vi "test1.vi"() -> ()   [LabVIEW 2022 SP3]
panel:
  out "String":string="import time\nimport ble_CBR\nimport bluetooth\nimport ble_advertising\nfrom ble_MIDI import *\nfrom hub import *\nimport device\nimport force_sensor\nimport distance_sensor\nimport motor\nimport color_sensor\nimport struct\nimport version\n\n\n#global\ndeviceTypeLookup = {48: 'm', 49: 'M', 61: 'Color S', 62: 'Distance S', 63: 'Force S', 255: 'N'}\nhubPorts = {'A': 'N', 'B': 'N', 'C': 'N', 'D': 'N', 'E': 'N', 'F': 'N'}\n\ndrumNotes = {31: 'Closed Hi-Hat', 32: 'Rim Shot', 33: 'Pedal Hi-Hat', 34: 'Snare Drum',\n    37: 'Side Stick', 39: 'Hand Clap', 41: 'Low Tom', 42: 'Closed Hi-Hat', 43: 'Low Tom',\n    44: 'Pedal Hi-Hat', 45: 'Mid Tom', 46: 'Open Hi-Hat', 47: 'Mid Tom', 48: 'High Tom',\n    49: 'Crash Cymbal', 50: 'High Tom', 51: 'Ride Cymbal', 52: 'Ride Cymbal', 53: 'Ride Bell',\n    54: 'Shaker', 57: 'Crash Cymbal', 59: 'Ride Cymbal', 86: 'Snare Drum', 90: 'Closed Hi-Hat',\n    91: 'Low Tom', 92: 'Closed Hi-Hat', 94: 'Pedal Hi-Hat', 95: 'Mid Tom',96: 'High Tom',\n    99: 'Ride Cymbal'}\n\n\n#initialize\nmidi = MIDI_Player('emma')\nmidi.wait_for_connection()\nPiano = MIDI_Instrument(midi, instruments['Acoustic Grand Piano'], channel=0)\n\n\n\n#firmware_check()\n\ndef done():\n    return button.pressed(button.RIGHT)\n\n\ndef test():\n    print(\"hi Emma!\")\n\n\ndef play_note(sensor, note, duration, dynamics = 'fff'):\n    \n    #print(\"in play_note\")\n\n    if type(note) == str:  \n        for key, value in drumNotes.items():\n            if value == note:\n                note = key  \n                #print(\"Found note:\", note)\n\n            \n    if (sensor == \"N\"):  \n        play_the_note(note, duration, dynamics)    \n        \n    elif (sensor == \"Force S\"):\n        if Force_Sensor_Activated():\n            play_the_note(note, duration, dynamics)\n        else:\n            print(\"waiing for FS activation\")\n            time.sleep(.1)\n            \n    elif (sensor == \"Color S\"):\n        if Color_Sensor_Activated():\n            play_the_note(note, duration, dynamics)\n        else:\n            print(\"waiting for CS activation\")\n            time.sleep(.1)\n            \n    elif (sensor == \"Distance S\"):\n        if Distance_Sensor_Activated():\n            the_port = check_port_connection(\"Distance S\")\n            dist = distance_sensor.distance(the_port)\n            dist_note = get_note_from_distance(dist)\n            play_the_note(dist_note, duration, dynamics)\n            #play_the_note(note, duration)\n        else:\n            print(\"waiting for DS activation\")\n            time.sleep(.1)\n            \n    elif ((sensor == \"m\") or (sensor == \"M\")):\n        #Need and if activated statment bc it could be not conencted\n        the_port = check_port_connection(sensor)\n        mpos = motor.absolute_position(the_port)\n    \n        if mpos < 0:\n            mpos = mpos + 360  \n        \n        print(mpos)\n        \n        note_range = 108 - 21  #Total number of notes in the range\n        note_value = int((mpos / 360) * note_range) + 21  #Maps the notes and value\n\n        play_the_note(note_value, .1, dynamics)\n        \n    else: \n        print(\"ELSE!!Invalid sensor type\")\n        time.sleep(.5)       \n\n\ndef play_chord(a, b=0, c=0, d=0, e=0, f=0, g=0, h=0):\n    Piano.on([a,b,c,d,e,f,g,h],velocity['f'])\n    time.sleep(.5)\n    Piano.off([a,b,c,d,e,f,g,h])\n        \n        \ndef play_the_note(note, duration, dynamics):\n    Piano.on(note, velocity[dynamics])\n    time.sleep(duration)\n    Piano.off(note, velocity[dynamics])\n\n\ndef Force_Sensor_Activated():\n    try:\n        the_port = check_port_connection(\"Force S\")\n        if the_port is None:\n            #print(\"Please connect the Force Sensor!\")\n            raise Exception(\"Force Sensor is NOT connected\")\n\n        if force_sensor.force(the_port) > 0:\n            print(\"Force Sensor is ACTIVATED\")\n            return True\n        else:\n            #print(\"FS FALSE\")\n            #time.sleep(.25)\n            return False\n    except Exception as e:\n        print(f\"Error: {e}\")\n        time.sleep(2)\n        return False\n    \ndef Color_Sensor_Activated():\n    try:\n        the_port = check_port_connection(\"Color S\")\n\n        if the_port is None:\n            #print(\"Please connect the Color Sensor!\")\n            raise Exception(\"Color Sensor is NOT connected\")\n\n        reflection = color_sensor.reflection(the_port)\n        if reflection > 50:\n            print(\"Color Sensor is ACTIVATED\")\n            return True\n        else:\n            return False\n    except Exception as e:\n        print(f\"Error: {e}\")\n        time.sleep(2)\n        return False\n    \n        \ndef Distance_Sensor_Activated():\n    try:\n        the_port = check_port_connection(\"Distance S\")\n        if the_port is None:\n            #print(\"Please connect the Distance Sensor!\")\n            raise Exception(\"Distance Sensor is NOT connected\")\n        \n        if distance_sensor.distance(the_port) > 0:\n            return True\n        else:\n            return False\n            \n    except Exception as e:\n        print(f\"Error: {e}\")\n        time.sleep(2)\n        return False    \n\n\n#def Motor_Activated():\n    \n\ndef disconnect():\n    print('disconnect')\n    midi.disconnect()\n\n\n\n\ndef NoteToNumber(note, octave = 0):\n    notes = {\"C\": 24,\"Db\": 25,\"D\": 26,\"Eb\": 27,\"E\": 28,\"F\": 29,\"Gb\": 30,\"G\": 31,\"Ab\": 32, \"A\": 33,\"Bb\": 34,\"B\": 35}\n    \n    try:  \n        if octave > 8 or octave < 0:\n            raise Exception(\"Invalid octave input\")\n        if note not in notes:\n            raise Exception(\"Invalid note input\")\n    \n        if(octave > 0):\n            return((notes[note]) + (octave*12))\n        \n    except Exception as e:\n        print(f\"Error: {e}\")\n        time.sleep(2)\n        return False\n        \n    \n'''-----Helper functions section (NOT intended for the user to use!)-----'''\n\ndef firmware_check():\n    try:\n        version.atlantis\n        print(version.atlantis)\n        print(\"Firmware is up to date! Good Job!\")\n    except:\n        print(\"Old Firmware: Please update your LEGO SPIKE hub to the latest firmware!\")\n\n\ndef get_note_from_distance(dist):\n    if dist == -1 or dist > 500:\n        return -1\n    elif dist < 500:\n        note = int(8 + (dist / 5))\n        return note\n\n\n\ndef ReadPorts():   \n    i = 0\n    for key in sorted(hubPorts): \n        hubPorts[key] = deviceTypeLookup.get(device.device_id(i))\n        i+=1\n            \n    return None\n\n\ndef is_connected(sensor):\n    ReadPorts()\n    \n    there_is_sensor = False\n    \n    i = 0\n    for port in sorted(hubPorts):\n        \n        if hubPorts[port] == sensor:\n            print(f\"{sensor} is connected to port.{port}\")\n            there_is_sensor = True\n    \n        if i == 5 and not there_is_sensor:\n            print(f\"{sensor} is NOT connected\")\n            print(\"--------------\")\n            raise ValueError(f\"{sensor} is not connected to any port\")\n            return False\n            \n        if i == 5 and there_is_sensor:\n            return True\n            \n        i+=1\n\n    return False\n\n\ndef check_port_connection(sensor):\n    ReadPorts()\n\n    i = 0\n    for port in sorted(hubPorts):\n        \n        if hubPorts[port] == sensor:\n            #print(\"connected\")\n            return string2port(f\"port.{port}\")\n            #return(f\"port.{port}\")\n    \n        if i == 5:\n            print(f\"{sensor} is NOT connected\")\n            print(\"--------------\")\n            #raise Exception(f\"{sensor} is NOT connected\")\n            return None\n    i+=1\n\n    return None\n        \n    \ndef string2port(portS):\n    if portS == \"port.A\": return port.A\n    if portS == \"port.B\": return port.B\n    if portS == \"port.C\": return port.C\n    if portS == \"port.D\": return port.D\n    if portS == \"port.E\": return port.E\n    if portS == \"port.F\": return port.F\n"
  out "number of replacements":i32
  out "result string":string
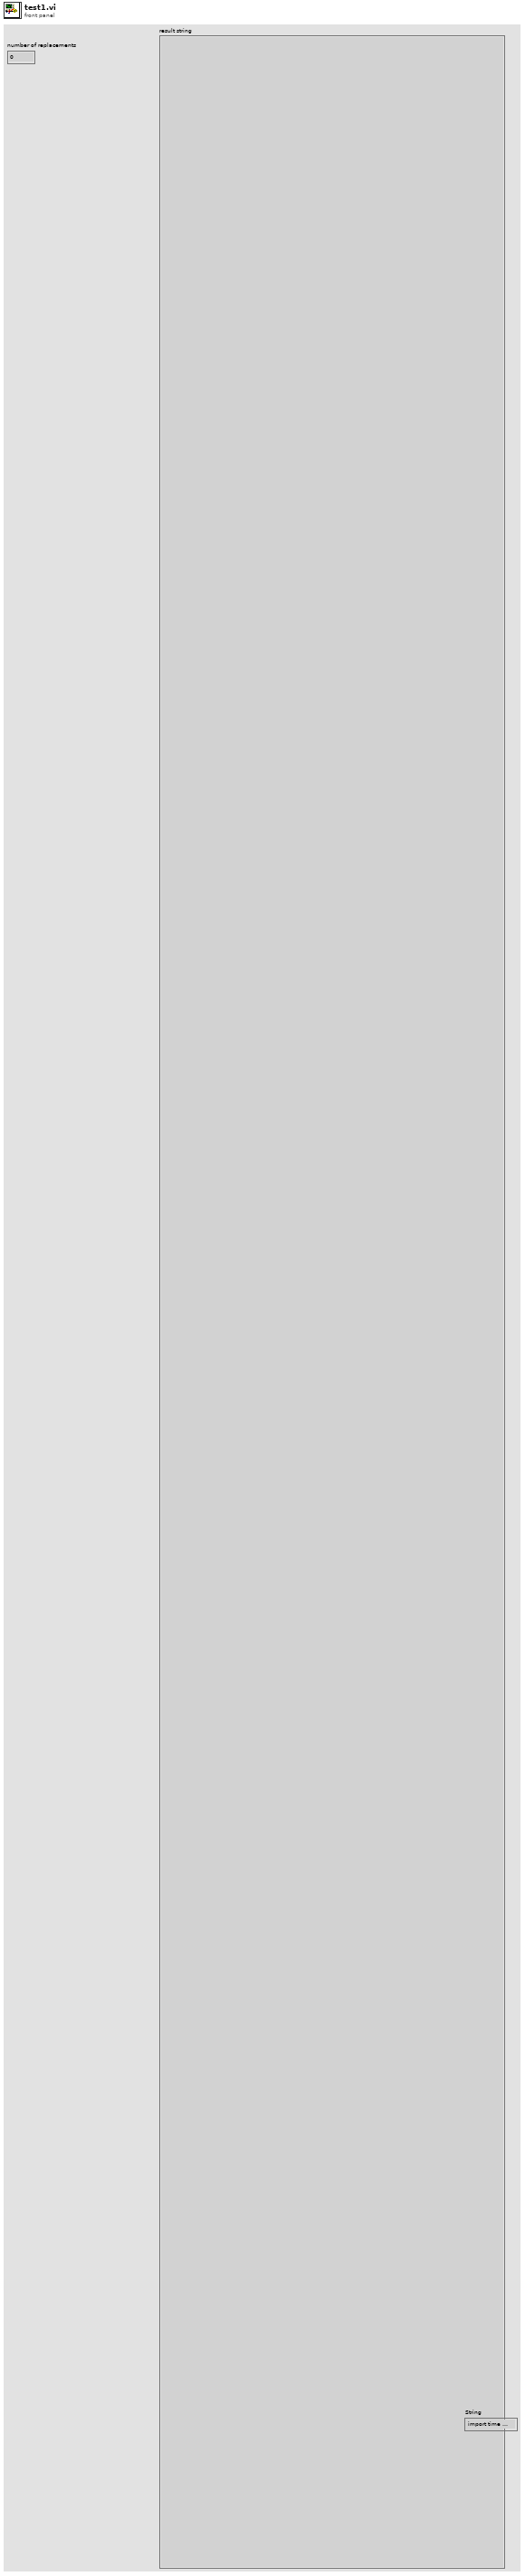
[diagram p1: front panel]
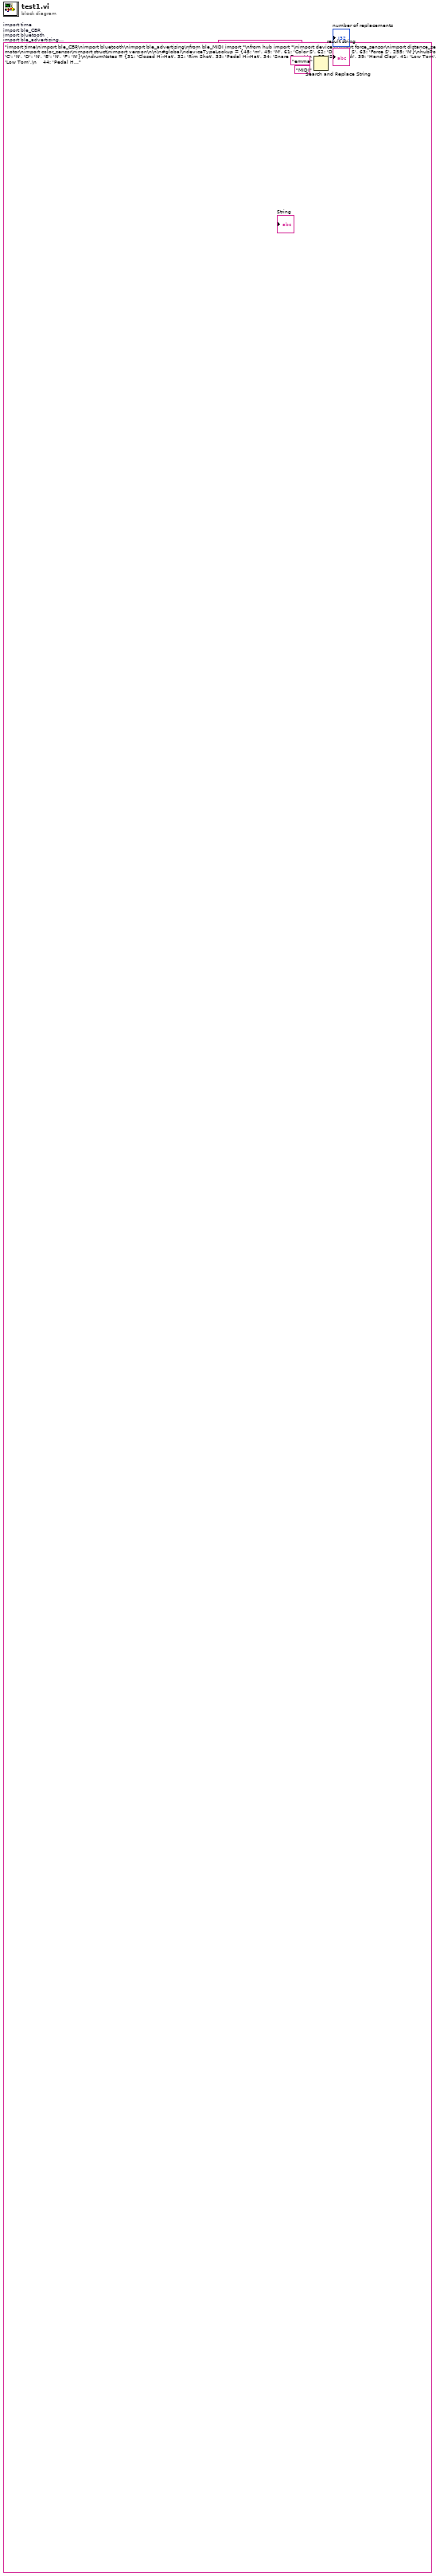
[diagram p0: block diagram]
diagram:
  w5 = "import time\nimport ble_CBR\nimport bluetooth\nimport ble_advertising\nfrom ble_MIDI import *\nfrom hub import *\nimport device\nimport force_sensor\nimport distance_sensor\nimport motor\nimport color_sensor\nimport struct\nimport version\n\n\n#global\ndeviceTypeLookup = {48: 'm', 49: 'M', 61: 'Color S', 62: 'Distance S', 63: 'Force S', 255: 'N'}\nhubPorts = {'A': 'N', 'B': 'N', 'C': 'N', 'D': 'N', 'E': 'N', 'F': 'N'}\n\ndrumNotes = {31: 'Closed Hi-Hat', 32: 'Rim Shot', 33: 'Pedal Hi-Hat', 34: 'Snare Drum',\n    37: 'Side Stick', 39: 'Hand Clap', 41: 'Low Tom', 42: 'Closed Hi-Hat', 43: 'Low Tom',\n    44: 'Pedal Hi-Hat', 45: 'Mid Tom', 46: 'Open Hi-Hat', 47: 'Mid Tom', 48: 'High Tom',\n    49: 'Crash Cymbal', 50: 'High Tom', 51: 'Ride Cymbal', 52: 'Ride Cymbal', 53: 'Ride Bell',\n    54: 'Shaker', 57: 'Crash Cymbal', 59: 'Ride Cymbal', 86: 'Snare Drum', 90: 'Closed Hi-Hat',\n    91: 'Low Tom', 92: 'Closed Hi-Hat', 94: 'Pedal Hi-Hat', 95: 'Mid Tom',96: 'High Tom',\n    99: 'Ride Cymbal'}\n\n\n#firmware_check()\n\ndef done():\n    return button.pressed(button.RIGHT)\n\n\ndef test():\n    print(\"hi Emma!\")\n\n\ndef play_note(sensor = \"N\", note = 60, duration = 1, dynamics = 'fff', port = None):\n    \n    #print(\"in play_note\")\n\n    if type(note) == str:  \n        for key, value in drumNotes.items():\n            if value == note:\n                note = key  \n                #print(\"Found note:\", note)\n\n            \n    if (sensor == \"N\"):  \n        play_the_note(note, duration, dynamics)    \n        \n    elif (sensor == \"Force S\"):\n        if Force_Sensor_Activated(port):\n            play_the_note(note, duration, dynamics)\n        else:\n            print(\"waiing for FS activation\")\n            time.sleep(.1)\n            \n    elif (sensor == \"Color S\"):\n        if Color_Sensor_Activated(port):\n            play_the_note(note, duration, dynamics)\n        else:\n            print(\"waiting for CS activation\")\n            time.sleep(.1)\n            \n    elif (sensor == \"Distance S\"):\n        if Distance_Sensor_Activated(port):\n            the_port = check_port_connection(\"Distance S\")\n            dist = distance_sensor.distance(the_port)\n            dist_note = get_note_from_distance(dist)\n            play_the_note(dist_note, duration, dynamics)\n            #play_the_note(note, duration)\n        else:\n            print(\"waiting for DS activation\")\n            time.sleep(.1)\n            \n    elif ((sensor == \"m\") or (sensor == \"M\")):\n        #Need and if activated statment bc it could be not conencted\n        the_port = check_port_connection(sensor)\n        mpos = motor.absolute_position(the_port)\n    \n        if mpos < 0:\n            mpos = mpos + 360  \n        \n        print(mpos)\n        \n        note_range = 108 - 21  #Total number of notes in the range\n        note_value = int((mpos / 360) * note_range) + 21  #Maps the notes and value\n\n        play_the_note(note_value, .1, dynamics)\n        \n    else: \n        print(\"ELSE!!Invalid sensor type\")\n        time.sleep(.5)       \n\n\ndef play_chord(a, b=0, c=0, d=0, e=0, f=0, g=0, h=0):\n    Piano.on([a,b,c,d,e,f,g,h],velocity['ff'])\n    time.sleep(.5)\n    Piano.off([a,b,c,d,e,f,g,h])\n        \n        \ndef play_the_note(note, duration, dynamics):\n    Piano.on(note, velocity[dynamics])\n    time.sleep(duration)\n    Piano.off(note, velocity[dynamics])\n\n\ndef Force_Sensor_Activated(port):\n    try:\n        if port is None:\n            the_ports = check_port_connection(\"Force S\")\n            if the_ports is None:\n                #print(\"Please connect the Force Sensor!\")\n                raise Exception(\"Force Sensor is NOT connected\")\n            \n            for port in the_ports:\n                if force_sensor.force(port) > 0:\n                    print(\"Force Sensor is ACTIVATED\")\n                    return True\n            \n            return False\n        else:\n            #print(\"Port was typed\") \n            if force_sensor.force(port) > 0:\n                print(\"Force Sensor is ACTIVATED\")\n                return True\n            else:\n                #print(\"FS FALSE\")\n                #time.sleep(.25)\n                return False\n                           \n    except Exception as e:\n        print(f\"Error: {e}\")\n        time.sleep(2)\n        return False\n\n\n    \ndef Color_Sensor_Activated(port):\n    try:\n        if port is None:\n            the_ports = check_port_connection(\"Color S\")\n            if the_ports is None:\n                #print(\"Please connect the Color Sensor!\")\n                raise Exception(\"Color Sensor is NOT connected\")\n            \n            for port in the_ports:\n                if color_sensor.reflection(port) > 50:\n                    print(\"Color Sensor is ACTIVATED\")\n                    return True\n            \n            return False\n        else:\n            if color_sensor.reflection(port) > 50:\n                print(\"Color Sensor is ACTIVATED\")\n                return True\n            else:\n                return False\n                \n    except Exception as e:\n        print(f\"Error: {e}\")\n        time.sleep(2)\n        return False\n  \n        \ndef Distance_Sensor_Activated(port):\n    try:\n        if port is None:\n            the_ports = check_port_connection(\"Distance S\")\n            if the_ports is None:\n                #print(\"Please connect the Color Sensor!\")\n                raise Exception(\"Distance Sensor is NOT connected\")\n            \n            for port in the_ports:\n                if distance_sensor.distance(the_port) > 0:\n                    print(\"Distance Sensor is ACTIVATED\")\n                    return True\n\n            return False\n        else:\n            if color_sensor.reflection(port) > 50:\n                print(\"Color Sensor is ACTIVATED\")\n                return True\n            else:\n                return False\n\n    except Exception as e:\n        print(f\"Error: {e}\")\n        time.sleep(2)\n        return False    \n\n\n#def Motor_Activated():\n    \n\ndef disconnect():\n    print('disconnect')\n    midi.disconnect()\n\n\n\n\ndef NoteToNumber(note, octave = 0):\n    notes = {\"C\": 24,\"Db\": 25,\"D\": 26,\"Eb\": 27,\"E\": 28,\"F\": 29,\"Gb\": 30,\"G\": 31,\"Ab\": 32, \"A\": 33,\"Bb\": 34,\"B\": 35}\n    \n    try:  \n        if octave > 8 or octave < 0:\n            raise Exception(\"Invalid octave input\")\n        if note not in notes:\n            raise Exception(\"Invalid note input\")\n    \n        if(octave > 0):\n            return((notes[note]) + (octave*12))\n        \n    except Exception as e:\n        print(f\"Error: {e}\")\n        time.sleep(2)\n        return False\n        \n    \n'''-----Helper functions section (NOT intended for the user to use!)-----'''\n\ndef firmware_check():\n    try:\n        version.atlantis\n        print(version.atlantis)\n        print(\"Firmware is up to date! Good Job!\")\n    except:\n        print(\"Old Firmware: Please update your LEGO SPIKE hub to the latest firmware!\")\n\n\ndef get_note_from_distance(dist):\n    if dist == -1 or dist > 500:\n        return -1\n    elif dist < 500:\n        note = int(8 + (dist / 5))\n        return note\n\n\n\ndef ReadPorts():   \n    i = 0\n    for key in sorted(hubPorts): \n        hubPorts[key] = deviceTypeLookup.get(device.device_id(i))\n        i+=1\n            \n    return None\n\n\ndef is_connected(sensor):\n    ReadPorts()\n    \n    there_is_sensor = False\n    \n    i = 0\n    for port in sorted(hubPorts):\n        \n        if hubPorts[port] == sensor:\n            print(f\"{sensor} is connected to port.{port}\")\n            there_is_sensor = True\n    \n        if i == 5 and not there_is_sensor:\n            print(f\"{sensor} is NOT connected\")\n            print(\"--------------\")\n            raise ValueError(f\"{sensor} is not connected to any port\")\n            return False\n            \n        if i == 5 and there_is_sensor:\n            return True\n            \n        i+=1\n\n    return False\n\n\ndef check_port_connection(sensor):\n    ReadPorts()\n    listOfPorts = []\n    is_a_connection = False\n    i = 0\n    for port in sorted(hubPorts):\n        \n        if hubPorts[port] == sensor:      \n            listOfPorts.append(string2port(f\"port.{port}\"))\n            is_a_connection = True\n            #return string2port(f\"port.{port}\")\n            #return(f\"port.{port}\")\n    \n        if i == 5 and is_a_connection:\n            #print(listOfPorts)\n            return listOfPorts\n            \n            \n        if i == 5 and not is_a_connection:\n            print(f\"{sensor} is NOT connected\")\n            print(\"--------------\")\n            #raise Exception(f\"{sensor} is NOT connected\")\n            return None\n        \n        i+=1\n    \n    return None\n        \n    \ndef string2port(portS):\n    if portS == \"port.A\": return port.A\n    if portS == \"port.B\": return port.B\n    if portS == \"port.C\": return port.C\n    if portS == \"port.D\": return port.D\n    if portS == \"port.E\": return port.E\n    if portS == \"port.F\": return port.F\n\n\n\n#initialize\nmidi = MIDI_Player('emma')\nmidi.wait_for_connection()\nPiano = MIDI_Instrument(midi, instruments['Acoustic Grand Piano'], channel=0)\n\n"  # import time import ble_CBR import bluetooth import ble_advertising from ble_MIDI import * from hub import * import device import force_sensor import distance_sensor import motor import color_sensor import struct import version   #global deviceTypeLookup = {48: 'm', 49: 'M', 61: 'Color S', 62: 'Distance S', 63: 'Force S', 255: 'N'} hubPorts = {'A': 'N', 'B': 'N', 'C': 'N', 'D': 'N', 'E': 'N', 'F': 'N'}  drumNotes = {31: 'Closed Hi-Hat', 32: 'Rim Shot', 33: 'Pedal Hi-Hat', 34: 'Snare Drum',     37: 'Side Stick', 39: 'Hand Clap', 41: 'Low Tom', 42: 'Closed Hi-Hat', 43: 'Low Tom',     44: 'Pedal Hi-Hat', 45: 'Mid Tom', 46: 'Open Hi-Hat', 47: 'Mid Tom', 48: 'High Tom',     49: 'Crash Cymbal', 50: 'High Tom', 51: 'Ride Cymbal', 52: 'Ride Cymbal', 53: 'Ride Bell',     54: 'Shaker', 57: 'Crash Cymbal', 59: 'Ride Cymbal', 86: 'Snare Drum', 90: 'Closed Hi-Hat',     91: 'Low Tom', 92: 'Closed Hi-Hat', 94: 'Pedal Hi-Hat', 95: 'Mid Tom',96: 'High Tom',     99: 'Ride Cymbal'}   #firmware_check()  def done():     return button.pressed(button.RIGHT)   def test():     print("hi Emma!")   def play_note(sensor = "N", note = 60, duration = 1, dynamics = 'fff', port = None):          #print("in play_note")      if type(note) == str:           for key, value in drumNotes.items():             if value == note:                 note = key                   #print("Found note:", note)                   if (sensor == "N"):           play_the_note(note, duration, dynamics)                  elif (sensor == "Force S"):         if Force_Sensor_Activated(port):             play_the_note(note, duration, dynamics)         else:             print("waiing for FS activation")             time.sleep(.1)                  elif (sensor == "Color S"):         if Color_Sensor_Activated(port):             play_the_note(note, duration, dynamics)         else:             print("waiting for CS activation")             time.sleep(.1)                  elif (sensor == "Distance S"):         if Distance_Sensor_Activated(port):             the_port = check_port_connection("Distance S")             dist = distance_sensor.distance(the_port)             dist_note = get_note_from_distance(dist)             play_the_note(dist_note, duration, dynamics)             #play_the_note(note, duration)         else:             print("waiting for DS activation")             time.sleep(.1)                  elif ((sensor == "m") or (sensor == "M")):         #Need and if activated statment bc it could be not conencted         the_port = check_port_connection(sensor)         mpos = motor.absolute_position(the_port)              if mpos < 0:             mpos = mpos + 360                    print(mpos)                  note_range = 108 - 21  #Total number of notes in the range         note_value = int((mpos / 360) * note_range) + 21  #Maps the notes and value          play_the_note(note_value, .1, dynamics)              else:          print("ELSE!!Invalid sensor type")         time.sleep(.5)          def play_chord(a, b=0, c=0, d=0, e=0, f=0, g=0, h=0):     Piano.on([a,b,c,d,e,f,g,h],velocity['ff'])     time.sleep(.5)     Piano.off([a,b,c,d,e,f,g,h])                   def play_the_note(note, duration, dynamics):     Piano.on(note, velocity[dynamics])     time.sleep(duration)     Piano.off(note, velocity[dynamics])   def Force_Sensor_Activated(port):     try:         if port is None:             the_ports = check_port_connection("Force S")             if the_ports is None:                 #print("Please connect the Force Sensor!")                 raise Exception("Force Sensor is NOT connected")                          for port in the_ports:                 if force_sensor.force(port) > 0:                     print("Force Sensor is ACTIVATED")                     return True                          return False         else:             #print("Port was typed")              if force_sensor.force(port) > 0:                 print("Force Sensor is ACTIVATED")                 return True             else:                 #print("FS FALSE")                 #time.sleep(.25)                 return False                                 except Exception as e:         print(f"Error: {e}")         time.sleep(2)         return False        def Color_Sensor_Activated(port):     try:         if port is None:             the_ports = check_port_connection("Color S")             if the_ports is None:                 #print("Please connect the Color Sensor!")                 raise Exception("Color Sensor is NOT connected")                          for port in the_ports:                 if color_sensor.reflection(port) > 50:                     print("Color Sensor is ACTIVATED")                     return True                          return False         else:             if color_sensor.reflection(port) > 50:                 print("Color Sensor is ACTIVATED")                 return True             else:                 return False                      except Exception as e:         print(f"Error: {e}")         time.sleep(2)         return False             def Distance_Sensor_Activated(port):     try:         if port is None:             the_ports = check_port_connection("Distance S")             if the_ports is None:                 #print("Please connect the Color Sensor!")                 raise Exception("Distance Sensor is NOT connected")                          for port in the_ports:                 if distance_sensor.distance(the_port) > 0:                     print("Distance Sensor is ACTIVATED")                     return True              return False         else:             if color_sensor.reflection(port) > 50:                 print("Color Sensor is ACTIVATED")                 return True             else:                 return False      except Exception as e:         print(f"Error: {e}")         time.sleep(2)         return False       #def Motor_Activated():       def disconnect():     print('disconnect')     midi.disconnect()     def NoteToNumber(note, octave = 0):     notes = {"C": 24,"Db": 25,"D": 26,"Eb": 27,"E": 28,"F": 29,"Gb": 30,"G": 31,"Ab": 32, "A": 33,"Bb": 34,"B": 35}          try:           if octave > 8 or octave < 0:             raise Exception("Invalid octave input")         if note not in notes:             raise Exception("Invalid note input")              if(octave > 0):             return((notes[note]) + (octave*12))              except Exception as e:         print(f"Error: {e}")         time.sleep(2)         return False               '''-----Helper functions section (NOT intended for the user to use!)-----'''  def firmware_check():     try:         version.atlantis         print(version.atlantis)         print("Firmware is up to date! Good Job!")     except:         print("Old Firmware: Please update your LEGO SPIKE hub to the latest firmware!")   def get_note_from_distance(dist):     if dist == -1 or dist > 500:         return -1     elif dist < 500:         note = int(8 + (dist / 5))         return note    def ReadPorts():        i = 0     for key in sorted(hubPorts):          hubPorts[key] = deviceTypeLookup.get(device.device_id(i))         i+=1                  return None   def is_connected(sensor):     ReadPorts()          there_is_sensor = False          i = 0     for port in sorted(hubPorts):                  if hubPorts[port] == sensor:             print(f"{sensor} is connected to port.{port}")             there_is_sensor = True              if i == 5 and not there_is_sensor:             print(f"{sensor} is NOT connected")             print("--------------")             raise ValueError(f"{sensor} is not connected to any port")             return False                      if i == 5 and there_is_sensor:             return True                      i+=1      return False   def check_port_connection(sensor):     ReadPorts()     listOfPorts = []     is_a_connection = False     i = 0     for port in sorted(hubPorts):                  if hubPorts[port] == sensor:                   listOfPorts.append(string2port(f"port.{port}"))             is_a_connection = True             #return string2port(f"port.{port}")             #return(f"port.{port}")              if i == 5 and is_a_connection:             #print(listOfPorts)             return listOfPorts                                   if i == 5 and not is_a_connection:             print(f"{sensor} is NOT connected")             print("--------------")             #raise Exception(f"{sensor} is NOT connected")             return None                  i+=1          return None               def string2port(portS):     if portS == "port.A": return port.A     if portS == "port.B": return port.B     if portS == "port.C": return port.C     if portS == "port.D": return port.D     if portS == "port.E": return port.E     if portS == "port.F": return port.F    #initialize midi = MIDI_Player('emma') midi.wait_for_connection() Piano = MIDI_Instrument(midi, instruments['Acoustic Grand Piano'], channel=0)
  n1 = Search and Replace String(input string=w5, search string="emma", replace string="MIDI" ("replace string (\"\")")) -> (result string=→"result string":string, number of replacements=→"number of replacements":i32)  [unwired: 5 in, 2 out]
  "String" <- w5
